vi "niRFUtil WFM Decimate Waveform (complex wfm).vi"(0 "Waveform In":T1 {"y" format="%.2f"; "dx" format="%^.2e"; "x0" format="%^.2e"}, 5 "Rate (1)":i32=1, 7 "Offset (0)":i32, 13 "Average? (F)":bool) -> (4 "Waveform Out":T1 {"y" format="%.2f"; "dx" format="%^.2e"; "x0" format="%^.2e"})   [LabVIEW 2015, in "niRFUtil.lvlib"]
doc: "(c) Copyright 2006, National Instruments, Inc. This VI may not be duplicated, sold, or distributed without written consent from National Instruments."
uses:
  niRFUtil.lvlib
  Includes/niRFUtil INC Complex Waveform.ctl
  Includes/niRFUtil INC Complex Array.ctl
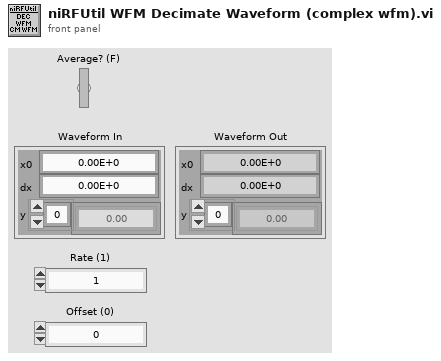
[diagram p1: front panel]
types:
  T1 = typedef "niRFUtil.lvlib/niRFUtil INC Complex Waveform.ctl" = cluster{"x0":dbl, "dx":dbl, "y":T2}
  T2 = typedef "niRFUtil.lvlib/niRFUtil INC Complex Array.ctl" = csg[]
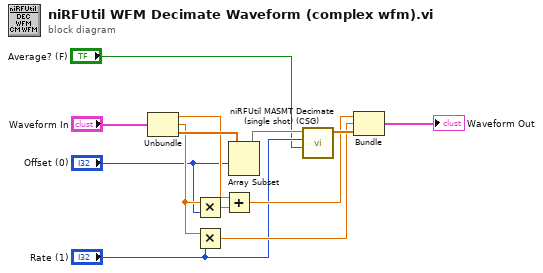
[diagram p0: block diagram]
diagram:
  n1 = Unbundle("Waveform In") -> ("x0"=w7:dbl, "dx"=w9:dbl, "y"=w12:T2)
  n2 = Multiply(x=w9, y="Offset (0)") -> (x*y=w8:dbl)
  n3 = Multiply(x=w9, y="Rate (1)") -> (x*y=w10:dbl)
  n4 = Add(x=w7, y=w8) -> (x+y=w6:dbl)
  n5 = Array Subset(array=w12, index="Offset (0)") -> (w13:T2)  [unwired: 1 in]
  n6 = call "niRFUtil MASMT Decimate (single shot) (CSG).vi"("averaging"="Average? (F)", "decimating factor"="Rate (1)", "X"=w13) -> ("Decimated X"=w11:csg[])  [unwired: 7 in, 1 out]
  n7 = Bundle(w6, w10, "Decimated X"=w11) -> (→"Waveform Out":cluster{dbl, dbl, "Decimated X":csg[]})  [unwired: 1 out]
